vi "Create Enum Getter.vi"(7 "RPC Message Name":string, 8 "error in (no error)":errorcluster, 11 "RPC Messages Folder (ProjectItem) in":refnum<vi>) -> (0 "error out":errorcluster, 2 "Message Getter out":refnum<vi>, 3 "RPC Messages Folder (ProjectItem) out":refnum<vi>)   [LabVIEW 2019, in "gRPC Template Creation Utility.lvlib"]
uses:
  gRPC Template Creation Utility.lvlib
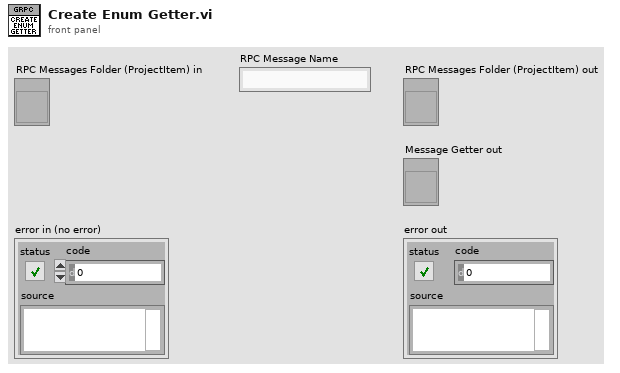
[diagram p1: front panel]
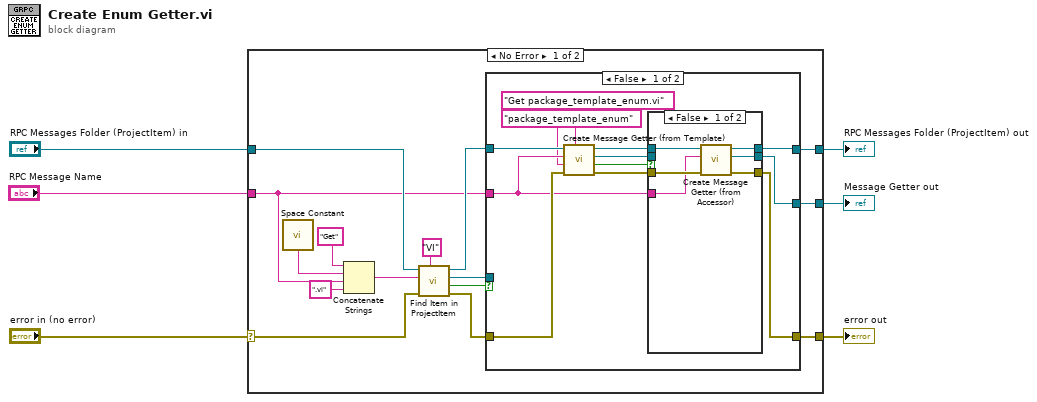
[diagram p0: block diagram]
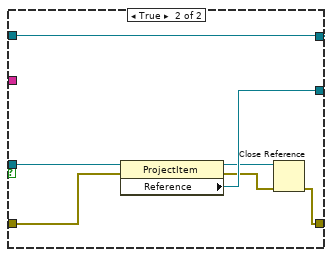
[diagram p3: hidden frame]
diagram:
  n1 = case shown="No Error" "error in (no error)" {
    selector: "error in (no error)" -> [w7 w51]
    tunnel: [w21 _] -> w6
    tunnel: [w20 w50] -> w5
    tunnel: [w19 w51] -> w4
    tunnel: "RPC Messages Folder (ProjectItem) in" -> [w17 w50]
    tunnel: "RPC Message Name" -> [w8 _]
    frame No Error {
      n2 = call <vilib>:"Space Constant.vi"() -> ("String"=w14:string)
      n3 = Concatenate Strings("Get" ("string"), w14, w8, ".vi" ("string")) -> (w12:string)
      n4 = call "Find Item in ProjectItem.vi"("Item Type"="VI", "error in (no error)"=w7, "Name"=w12, "ProjectItem in"=w17) -> ("error out"=w10:errorcluster, "Found ?"=w11:bool, "Item Refnum out"=w9:refnum<vi>, "ProjectItem out"=w16:refnum<vi>)  [unwired: 4 in]
      n5 = case shown="False" w11 {
        tunnel: [w24 w48] -> w21
        tunnel: [w27 w47] -> w20
        tunnel: w10 -> [w33 w44]
        tunnel: [w25 w43] -> w19
        tunnel: w16 -> [w32 w47]
        tunnel: w9 -> [_ w49]
        tunnel: w8 -> [w26 _]
        frame False {
          n6 = call "Create Message Getter (from Template).vi"("replace string in template"="package_template_enum", "error in (no error)"=w33, "template VI name"="Get package_template_enum.vi", "RPC Message Name"=w26, "RPC Messages Folder (ProjectItem) in"=w32) -> ("error out"=w30:errorcluster, "Created?"=w31:bool, "Getter VI out"=w28:refnum<vi>, "RPC Messages Folder (ProjectItem) out"=w29:refnum<vi>)  [unwired: 3 in]
          n7 = case shown="False" w31 {
            tunnel: w30 -> [w39 w41]
            tunnel: w29 -> [w38 w42]
            tunnel: w28 -> [_ w40]
            tunnel: [w35 w42] -> w27
            tunnel: [w36 w41] -> w25
            tunnel: [w34 w40] -> w24
            tunnel: w26 -> [w37 _]
            frame False {
              n8 = call "Create Message Getter (from Accessor).vi"("error in (no error)"=w39, "RPC Message Name"=w37, "RPC Messages Folder (ProjectItem) in"=w38) -> ("error out"=w36:errorcluster, "Getter VI out"=w34:refnum<vi>, "RPC Messages Folder (ProjectItem) out"=w35:refnum<vi>)  [unwired: 5 in, 1 out]
            }
            frame True {
            }
          }
        }
        frame True {
          n9 = property class="ProjectItem"(reference=w49, error in=w44) -> (reference out=w45:refnum<vi>, error out=w46:errorcluster, "Reference"=w48:refnum<vi>)
          n10 = Close Reference(reference=w45, error in (no error)=w46) -> (error out=w43:errorcluster)
        }
      }
    }
    frame Error {
    }
  }
  "error out" <- w4
  "Message Getter out" <- w6
  "RPC Messages Folder (ProjectItem) out" <- w5
